vi "Prime BSI R3 Camera Messenger.vi"(0 "Notifier Name":string, 2 "Prime Actions":T5, 5 "Prime Parameter":T2, 7 "ROI Setup":T1, 9 "# of Frames":u32, 11 "File Save Path":path) -> (4 "Notifier Name (Dup)":string, 6 "Prime Parameter":T2, 8 "Prime ROI":T1, 10 "Running?":bool, 13 "Image Ref":T4, 15 "Error?":bool)   [LabVIEW 2016]
uses:
  Prime BSI R3 Controls/Prime R3 Actions.ctl
  Prime BSI R3 Controls/Prime R3 Parameters.ctl
  Prime BSI R3 Controls/Prime R3 Parameter List.ctl
  Prime BSI R3 Controls/Prime R3 ROI.ctl
  <vilib>/vision/Image Controls.llb/IMAQ Image.ctl
  Prime BSI R3 Controls/Prime R3 Notifier Element.ctl
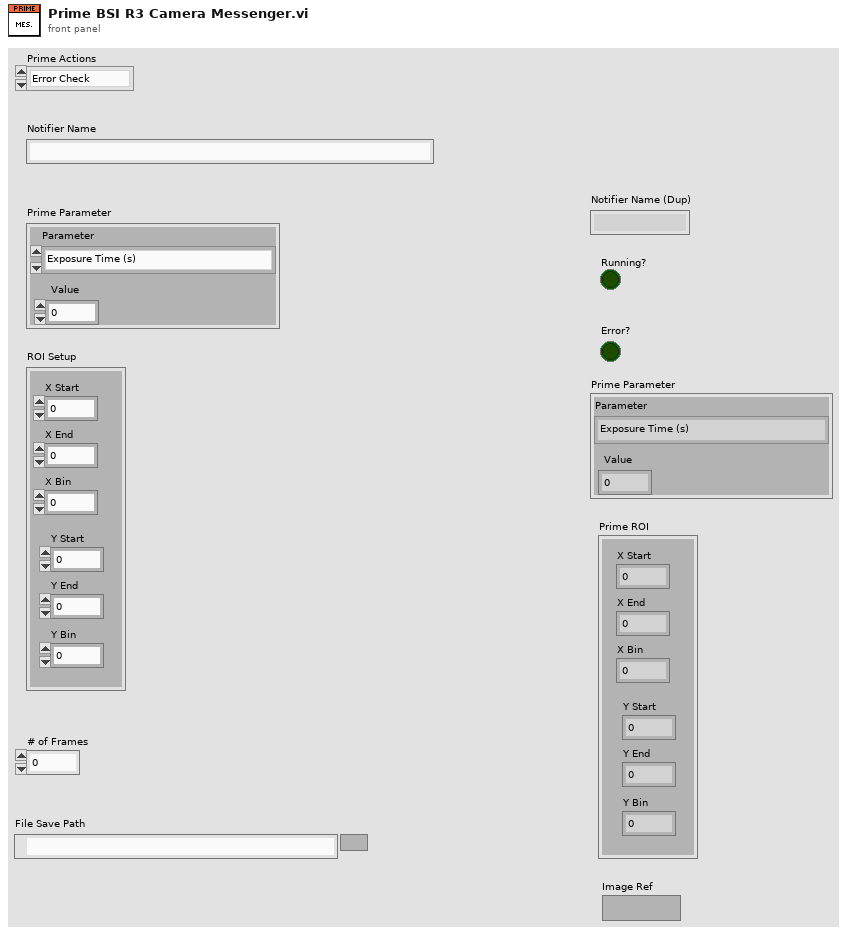
[diagram p1: front panel]
types:
  T1 = typedef "Prime R3 ROI.ctl" = cluster{"X Start":u32, "X End":u32, "X Bin":u32, "Y Start":u32, "Y End":u32, "Y Bin":u32}
  T2 = typedef "Prime R3 Parameters.ctl" = cluster{"Parameter":T3, "Value":dbl}
  T3 = typedef "Prime R3 Parameter List.ctl" = enum16{"Exposure Time (s)"}
  T4 = typedef "IMAQ Image.ctl" = refnum<image>
  T5 = typedef "Prime R3 Actions.ctl" = enum16{"Error Check", "Initialize", "Preview", "Record", "Abort", "Record Settings", "Set Parameter", "Get Parameter", "Set ROI", "Get ROI", "Status", "Set Trigger", "Quit"}
  T6 = typedef "Prime R3 Notifier Element.ctl" = cluster{"Prime Actions":T5, "Received?":bool, "Prime Parameter":T2, "Prime ROI":T1, "Running?":bool, "File Path":path, "# of frames":u32, "Image Ref":T4, "Error":errorcluster}
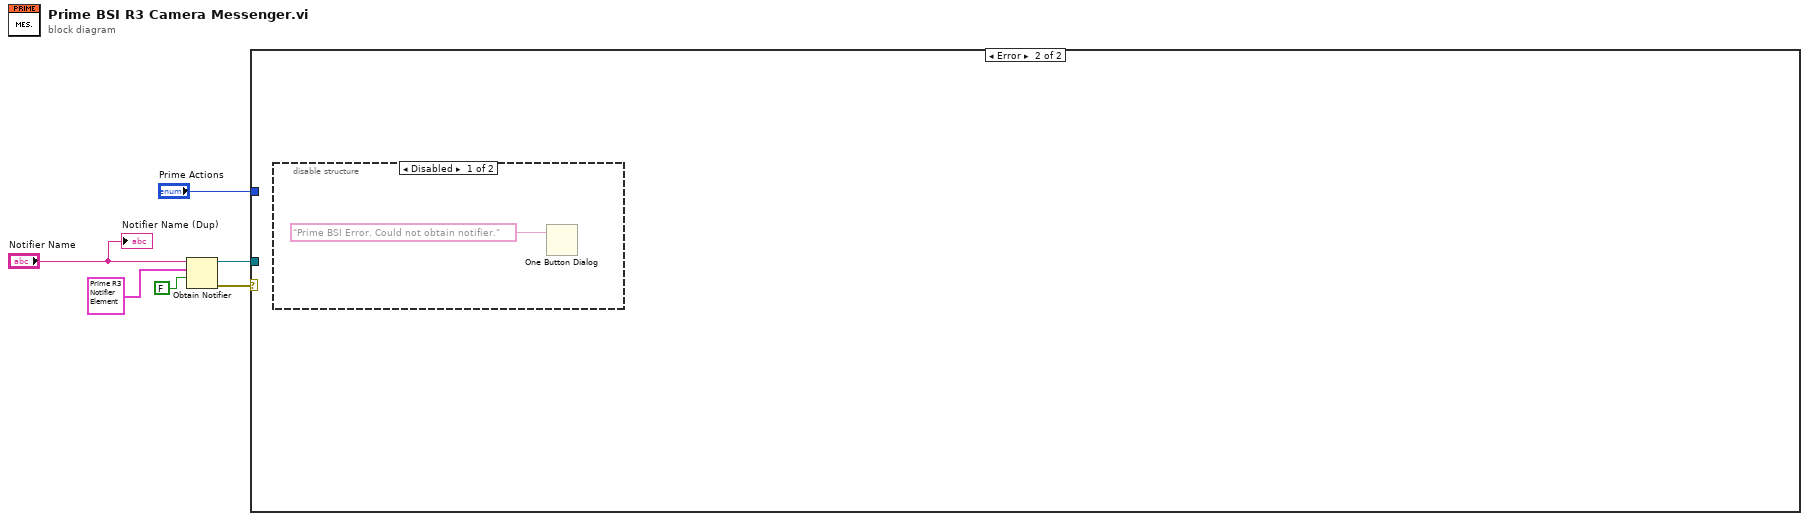
[diagram p0: block diagram]
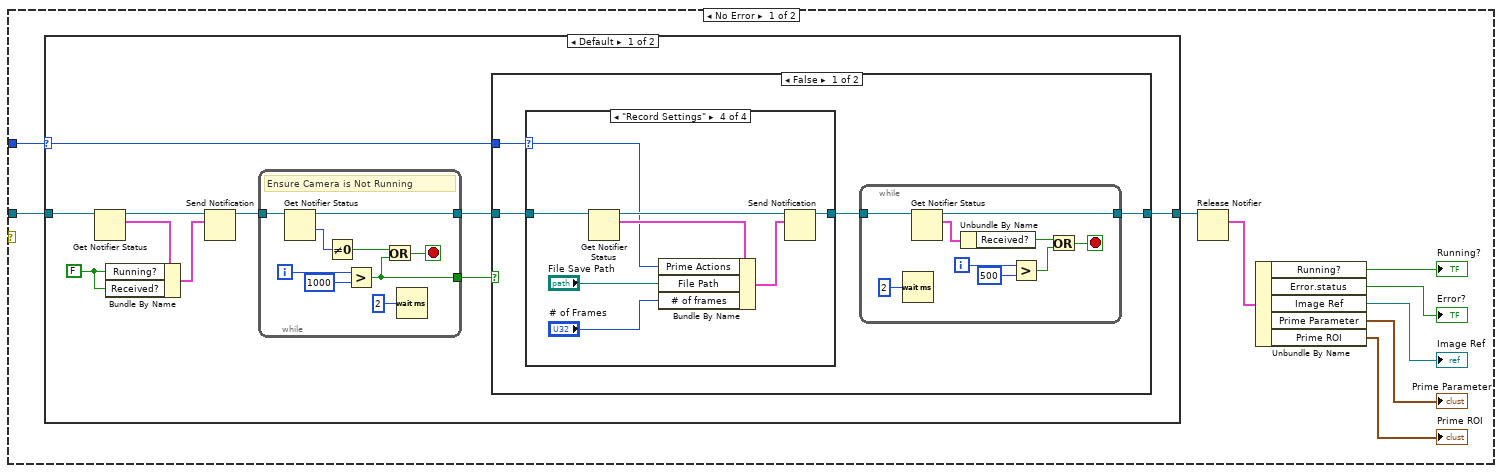
[diagram p2: hidden frame]
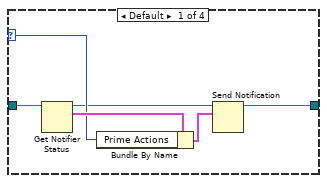
[diagram p3: hidden frame]
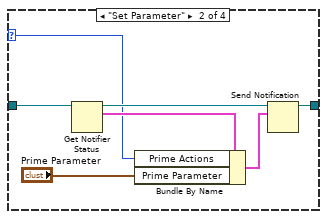
[diagram p4: hidden frame]
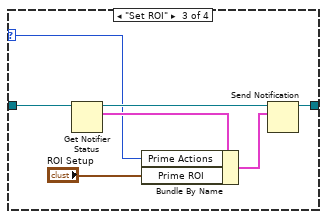
[diagram p5: hidden frame]
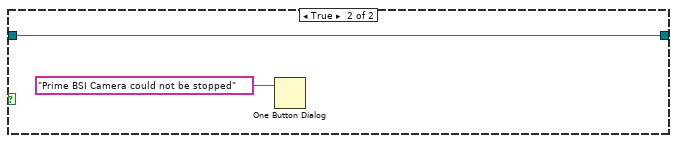
[diagram p6: hidden frame]
diagram:
  n1 = Obtain Notifier(name (unnamed)="Notifier Name", notification data type=T6 {"Prime Actions"=enum."Error Check", "Received?"=FALSE, "Prime Parameter"={"Parameter"=enum."Exposure Time (s)", "Value"=0.0}, "Prime ROI"={"X Start"=0, "X End"=0, "X Bin"=0, "Y Start"=0, "Y End"=0, "Y Bin"=0}, "Running?"=FALSE, "File Path"=path "", "# of frames"=0, "Image Ref"=refnum, "Error"={"status"=FALSE, "code"=0, "source"=""}} ("Prime Camera Cluster"), create if not found? (T)=FALSE) -> (notifier out=w4:refnum<notifier>, error out=w5:errorcluster)  [unwired: 1 in, 1 out]
  n2 = case shown="Error" w5 {
    tunnel: w4 -> [w15 _]
    tunnel: "Prime Actions" -> [w14 _]
    frame No Error {
      n3 = case shown="Default" w14 {
        selector: w14 -> [w21 _]
        tunnel: w15 -> [w25 w78]
        tunnel: [w20 w78] -> w8
        frame Default {
          w16 = FALSE ("Running?")
          n4 = Get Notifier Status(notifier=w25) -> (notifier out=w19:refnum<notifier>, current notification=w18:T6)  [unwired: 1 in, 3 out]
          n5 = Bundle By Name(cluster=w18, "Running?"=w16, "Received?"=w16) -> (w17:T6)
          n6 = Send Notification(notification=w17, notifier=w19) -> (notifier out=w24:refnum<notifier>)  [unwired: 1 in, 1 out]
          n7 = while {
            tunnel: w24 -> [w77]
            tunnel: [w76] -> w22
            tunnel: [w71] -> w23
            i -> [w73]
            stop <- w75 stop-if-true
            # "Ensure Camera is Not Running"
            n8 = Get Notifier Status(notifier=w77) -> (notifier out=w76:refnum<notifier>, # waiting=w70:i32)  [unwired: 1 in, 3 out]
            n9 = Not Equal To 0?(x=w70) -> (x != 0?=w69:bool)
            n10 = Greater?(x=w73, y=1000) -> (0:w71:bool)
            n11 = Or(x=w69, y=w71) -> (x .or. y?=w75:bool)
            n12 = Wait (ms)(milliseconds to wait=u32 2) -> ()  [unwired: 1 out]
          }
          n13 = case shown="False" w23 {
            tunnel: w22 -> [w27 w67]
            tunnel: w21 -> [w29 _]
            tunnel: [w26 w67] -> w20
            frame False {
              n14 = case shown="\"Record Settings\"" w29 {
                selector: w29 -> [w42 w46 w53 w61]
                tunnel: w27 -> [w44 w51 w58 w66]
                tunnel: [w39 w49 w56 w64] -> w28
                frame Default {
                  n15 = Get Notifier Status(notifier=w44) -> (notifier out=w41:refnum<notifier>, current notification=w43:T6)  [unwired: 1 in, 3 out]
                  n16 = Bundle By Name(cluster=w43, "Prime Actions"=w42) -> (w40:T6)
                  n17 = Send Notification(notification=w40, notifier=w41) -> (notifier out=w39:refnum<notifier>)  [unwired: 1 in, 1 out]
                }
                frame "Set Parameter" {
                  n18 = Get Notifier Status(notifier=w51) -> (notifier out=w50:refnum<notifier>, current notification=w48:T6)  [unwired: 1 in, 3 out]
                  n19 = Bundle By Name(cluster=w48, "Prime Actions"=w46, "Prime Parameter"="Prime Parameter") -> (w47:T6)
                  n20 = Send Notification(notification=w47, notifier=w50) -> (notifier out=w49:refnum<notifier>)  [unwired: 1 in, 1 out]
                }
                frame "Set ROI" {
                  n21 = Get Notifier Status(notifier=w58) -> (notifier out=w57:refnum<notifier>, current notification=w55:T6)  [unwired: 1 in, 3 out]
                  n22 = Bundle By Name(cluster=w55, "Prime Actions"=w53, "Prime ROI"="ROI Setup") -> (w54:T6)
                  n23 = Send Notification(notification=w54, notifier=w57) -> (notifier out=w56:refnum<notifier>)  [unwired: 1 in, 1 out]
                }
                frame "Record Settings" {
                  n24 = Get Notifier Status(notifier=w66) -> (notifier out=w65:refnum<notifier>, current notification=w63:T6)  [unwired: 1 in, 3 out]
                  n25 = Bundle By Name(cluster=w63, "Prime Actions"=w61, "File Path"="File Save Path", "# of frames"="# of Frames") -> (w62:T6)
                  n26 = Send Notification(notification=w62, notifier=w65) -> (notifier out=w64:refnum<notifier>)  [unwired: 1 in, 1 out]
                }
              }
              n27 = while {
                tunnel: w28 -> [w38]
                tunnel: [w30] -> w26
                i -> [w35]
                stop <- w31 stop-if-true
                n28 = Wait (ms)(milliseconds to wait=u32 2) -> ()  [unwired: 1 out]
                n29 = Get Notifier Status(notifier=w38) -> (notifier out=w30:refnum<notifier>, current notification=w37:T6)  [unwired: 1 in, 3 out]
                n30 = Unbundle By Name(w37) -> ("Received?"=w36:bool)
                n31 = Greater?(x=w35, y=500) -> (0:w33:bool)
                n32 = Or(x=w36, y=w33) -> (x .or. y?=w31:bool)
              }
            }
            frame True {
              n33 = One Button Dialog(message="Prime BSI Camera could not be stopped") -> ()  [unwired: 1 in, 1 out]
            }
          }
        }
        frame "Status" {
        }
      }
      n34 = Release Notifier(notifier=w8) -> (last notification=w7:T6)  [unwired: 2 in, 2 out]
      n35 = Unbundle By Name(w7) -> ("Running?"=→"Running?":bool, "Error.status"=→"Error?":bool, "Image Ref"=→"Image Ref":T4, "Prime Parameter"=→"Prime Parameter":T2, "Prime ROI"=→"Prime ROI":T1)
    }
    frame Error {
      n36 = disable-structure shown="Disabled" {
        frame Disabled {
          n37 = One Button Dialog(message="Prime BSI Error. Could not obtain notifier.") -> ()  [unwired: 1 in, 1 out]
        }
        frame Enabled {
        }
      }
    }
  }
  "Notifier Name (Dup)" <- "Notifier Name"
